vi "2B_Data_Split.vi"(7 "Input data":string, 11 "error in":errorcluster) -> (4 "Unix Time":string, 8 "Data String":string, 15 "error out":errorcluster)   [LabVIEW 2012]
uses:
  <vilib>/Utility/error.llb/whitespace.ctl
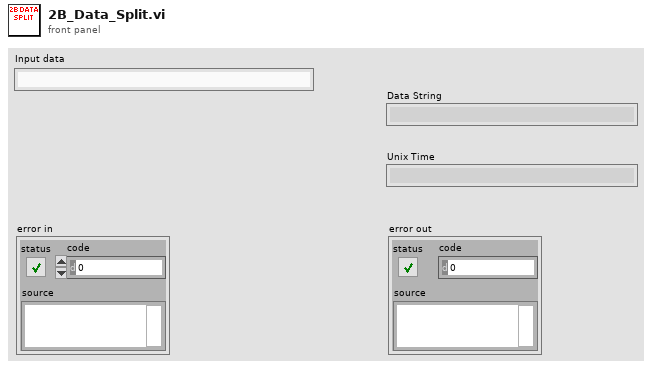
[diagram p1: front panel]
types:
  T1 = typedef "whitespace.ctl" = u16
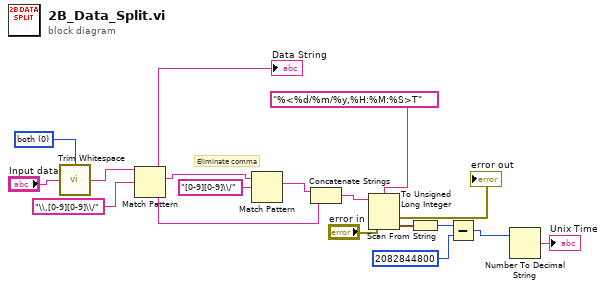
[diagram p0: block diagram]
diagram:
  w8 = T1 0 items=["both", "start of string", "end of string"] ("location (both)")
  # "Eliminate comma"
  n1 = call <vilib>:"Trim Whitespace.vi"("string"="Input data", "location (both)"=w8) -> ("trimmed string"=w6:string)
  n2 = Match Pattern(string=w6, regular expression="\\,[0-9][0-9]\\/") -> (before substring=→"Data String":string, match substring=w3:string, after substring=w4:string)  [unwired: 1 in, 1 out]
  n3 = Match Pattern(string=w3, regular expression="[0-9][0-9]\\/") -> (match substring=w1:string)  [unwired: 1 in, 3 out]
  n4 = Concatenate Strings(w1, w4) -> (w17:string)
  n5 = Scan From String(format string="%<%d/%m/%y,%H:%M:%S>T", input string=w17, error in="error in") -> (error out=→"error out":errorcluster, output 1=w16:timestamp)  [unwired: 2 in, 2 out]
  n6 = To Unsigned Long Integer(number=w16) -> (unsigned 32bit integer=w15:u32)
  n7 = Subtract(x=w15, y=u32 2082844800) -> (x-y=w11:u32)
  n8 = Number To Decimal String(number=w11) -> (decimal integer string=→"Unix Time":string)  [unwired: 1 in]
